vi "Format Body.vi"(4 "Indent":string, 6 "Name":string, 7 "Meta Data":string, 8 "Header":string, 9 "Attributes":string, 10 "Body":string, 11 "XML in":refnum<class "XML.lvclass">) -> (1 "String out":string, 3 "XML out":refnum<class "XML.lvclass">)   [LabVIEW 2020, in "XML.lvlib" / "XML.lvclass"]
uses:
  <vilib>/gpm_packages/@cs/persistence/source/XML/XML.lvclass
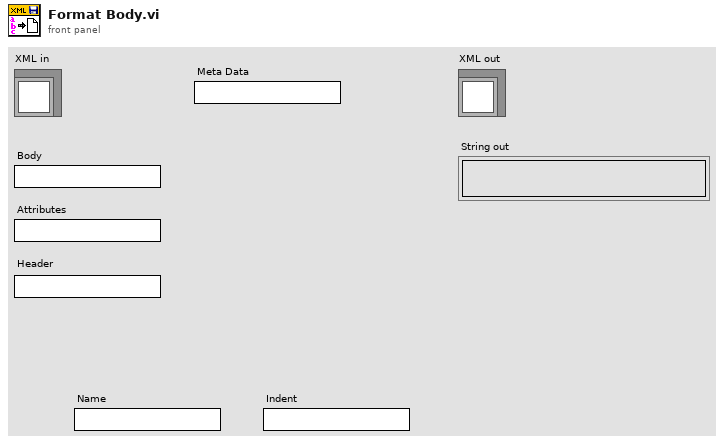
[diagram p1: front panel]
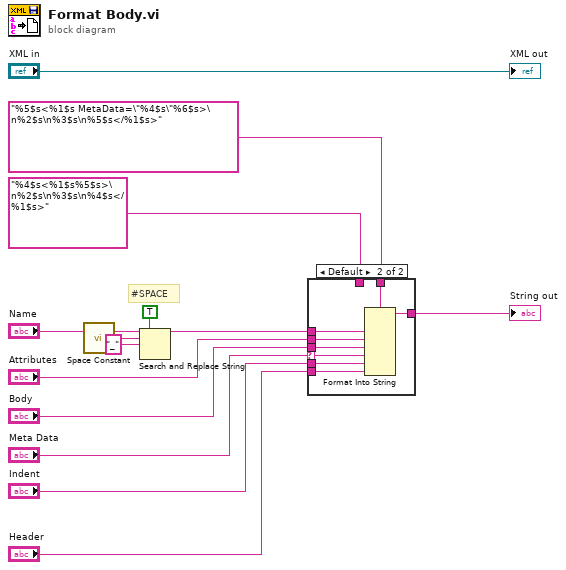
[diagram p0: block diagram]
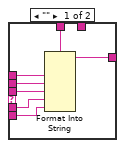
[diagram p2: hidden frame]
diagram:
  # "#SPACE"
  n1 = call <vilib>:"Space Constant.vi"() -> ("String"=w13:string)
  n2 = Search and Replace String(replace all?=TRUE ("replace all? (F)"), input string="Name", search string=w13, replace string="_") -> (result string=w7:string)  [unwired: 4 in, 3 out]
  n3 = case shown="Default" "Meta Data" {
    selector: "Meta Data" -> [_ w25]
    tunnel: [w17 w29] -> w6
    tunnel: "Body" -> [w19 w28]
    tunnel: "Attributes" -> [w20 w27]
    tunnel: w7 -> [w21 w26]
    tunnel: "%5$s<%1$s MetaData=\"%4$s\"%6$s>\n%2$s\n%3$s\n%5$s</%1$s>" ("format string") -> [_ w24]
    tunnel: "%4$s<%1$s%5$s>\n%2$s\n%3$s\n%4$s</%1$s>" ("format string") -> [w18 _]
    tunnel: "Indent" -> [w15 w23]
    tunnel: "Header" -> [w16 w22]
    frame "" {
      n4 = Format Into String(format string=w18, w21, w20, w19, w15, w16) -> (resulting string=w17:string)  [unwired: 2 in, 1 out]
    }
    frame Default {
      n5 = Format Into String(format string=w24, w26, w27, w28, w25, w23, w22) -> (resulting string=w29:string)  [unwired: 2 in, 1 out]
    }
  }
  "String out" <- w6
  "XML out" <- "XML in"
